vi "Rolling Average.vi"(9 "Enum":enum16{"Average", "Init"}(ring)=enum."Init", 10 "Value":dbl, 11 "Samples to Average":i32=100) -> (1 "mean":dbl)   [LabVIEW 2010]
uses:
  <vilib>/Analysis/NI_AALBase.lvlib
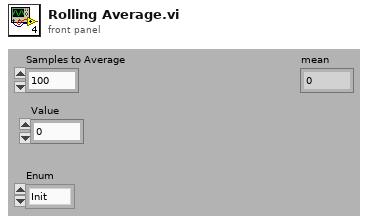
[diagram p1: front panel]
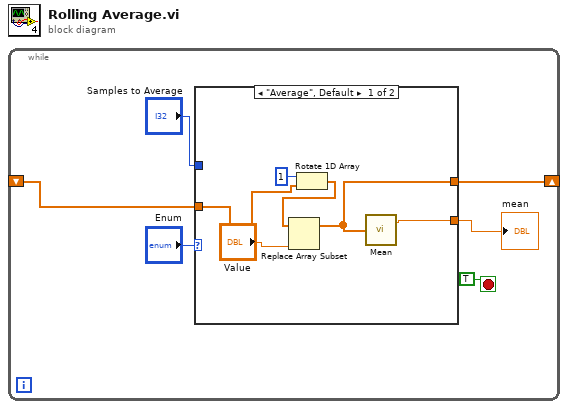
[diagram p0: block diagram]
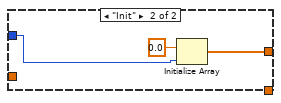
[diagram p2: hidden frame]
diagram:
  n1 = while {
    shift-right: [w4] -> _
    shift-left: _ -> [w6]
    stop <- TRUE stop-if-true
    n2 = case shown="\"Average\", Default" "Enum" {
      tunnel: w6 -> [w9 _]
      tunnel: "Samples to Average" -> [_ w13]
      tunnel: [w12 _] -> w1
      tunnel: [w7 w14] -> w4
      frame "Average", Default {
        n3 = Rotate 1D Array(1:w9, 2:1 ("n")) -> (0:w8:dbl[])
        n4 = Replace Array Subset(array=w8, new element="Value") -> (w7:dbl[])  [unwired: 1 in]
        n5 = call <vilib>:"Mean.vi"("X"=w7) -> ("mean"=w12:dbl)  [unwired: 1 out]
      }
      frame "Init" {
        n6 = Initialize Array(0.0 ("element"), w13) -> (w14:dbl[])
      }
    }
    "mean" <- w1
  }
